vi "CommandDynamixelPositionNoNotifiers.vi"(6 "NotifierReff":T1, 7 "Dynamixel Bounds":T4={"Main Dynamixel Set Data"={"Lower Winch Bound (deg)"=0.0, "Upper Winch Bound (deg)"=800.0}, "Rudder Dynamixel Set Data"={"Lower Winch Bound (deg)"=0.0, "Upper Winch Bound (deg)"=30.0}, "Jib Dynamixel Set Data"={"Lower Winch Bound (deg)"=0.0, "Upper Winch Bound (deg)"=800.0}}, 8 "error in":errorcluster, 9 "FPGA VI Reference In":refnum<k20>, 10 "Dynamixel Cycles":T3, 11 "VISA resource name":refnum<visa-resource-name>) -> (0 "Error out":errorcluster, 2 "Commanded rudder value":T2 min=-0.95 max=0.95 scale=1.0..-1.0, 3 "Debug sail value":dbl, 5 "VISA resource name OUT":refnum<visa-resource-name>)   [LabVIEW 2013]
doc: "First thing to know is that there is a boolean detection switch in this VI that you can switch between RC testing and code control.\n\nWhen RC testing, this VI checks the FPGA for RC data, bounds it so that the data is from 0-1 in steps of 0.05, converts that 0-1 value (or -1 to 1 for the rudder) into Dynamixel degrees (1200 dynamixel counts per 360 degrees) and then writes that position to the Dynamixel. This is highly dependent on the motor bounds which are passed in from above, because a sail value of 1 means different things when the motor bounds are different.\n\nCode control takes the notifier with sail/rudder positions and commands those positions.\n\nEric Schneider, October 2014"
uses:
  Data/TypeDefs/MotorSetup.ctl
  Data/TypeDefs/DynamixelSetupInfo.ctl
  Data/TypeDefs/DynamixelCycleTracker.ctl
  Data/TypeDefs/Rudder Set Suggestions.ctl
  Data/TypeDefs/Notifiers.ctl
  Data/TypeDefs/UTM Location.ctl
  Data/TypeDefs/Sail Set Suggestions.ctl
  Data/TypeDefs/OverrideInformation.ctl
  Data/TypeDefs/OverrideMode.ctl
  Data/TypeDefs/AirmarStatus.ctl
  Data/TypeDefs/HardwareOnline.ctl
  Data/TypeDefs/RC Input Values.ctl
  Classes/Waypoint/Waypoint.lvclass
panel:
  out "Use RC Control?":bool
  out "Rudder written value":dbl
  out "Main written value":dbl
  out "Jib written value":dbl
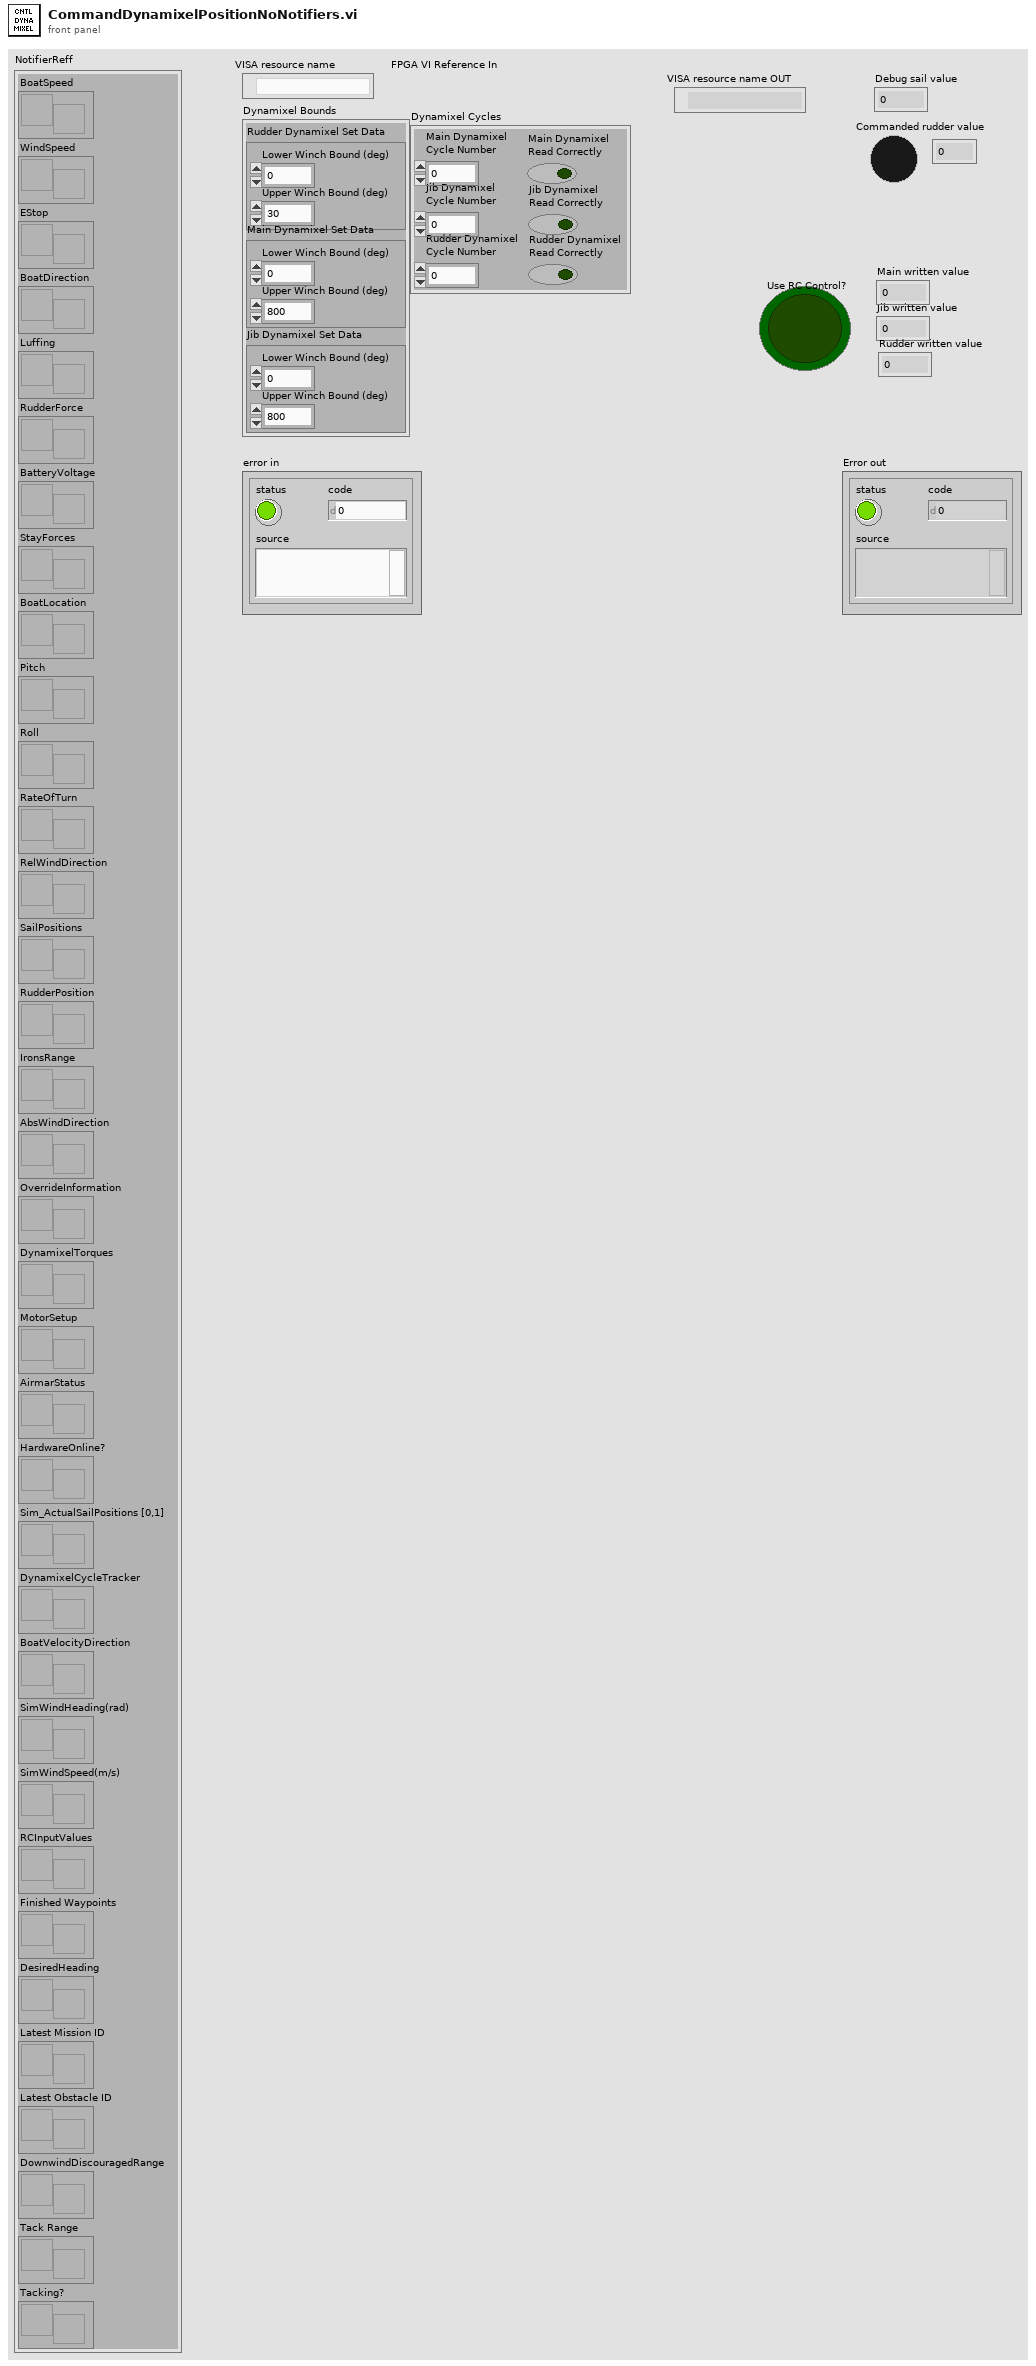
[diagram p1: front panel]
types:
  T1 = typedef "Notifiers.ctl" = cluster{"BoatSpeed":refnum<notifier>, "WindSpeed":refnum<notifier>, "EStop":refnum<notifier>, "BoatDirection":refnum<notifier>, "Luffing":refnum<notifier>, "RudderForce":refnum<notifier>, "BatteryVoltage":refnum<notifier>, "StayForces":refnum<notifier>, "BoatLocation":refnum<notifier>, "Pitch":refnum<notifier>, "Roll":refnum<notifier>, "RateOfTurn":refnum<notifier>, "RelWindDirection":refnum<notifier>, "SailPositions":refnum<notifier>, "RudderPosition":refnum<notifier>, "IronsRange":refnum<notifier>, "AbsWindDirection":refnum<notifier>, "OverrideInformation":refnum<notifier>, "DynamixelTorques":refnum<notifier>, "MotorSetup":refnum<notifier>, "AirmarStatus":refnum<notifier>, "HardwareOnline?":refnum<notifier>, "Sim_ActualSailPositions [0,1]":refnum<notifier>, "DynamixelCycleTracker":refnum<notifier>, "BoatVelocityDirection":refnum<notifier>, "SimWindHeading(rad)":refnum<notifier>, "SimWindSpeed(m/s)":refnum<notifier>, "RCInputValues":refnum<notifier>, "Finished Waypoints":refnum<notifier>, "DesiredHeading":refnum<notifier>, "Latest Mission ID":refnum<notifier>, "Latest Obstacle ID":refnum<notifier>, "DownwindDiscouragedRange":refnum<notifier>, "Tack Range":refnum<notifier>, "Tacking?":refnum<notifier>}
  T2 = typedef "Rudder Set Suggestions.ctl" = dbl
  T3 = typedef "DynamixelCycleTracker.ctl" = cluster{"Main Dynamixel\nCycle Number":i32, "Jib Dynamixel\nCycle Number":i32, "Rudder Dynamixel\nCycle Number":i32, "Main Dynamixel\nRead Correctly":bool, "Jib Dynamixel\nRead Correctly":bool, "Rudder Dynamixel\nRead Correctly":bool}
  T4 = typedef "MotorSetup.ctl" = cluster{"Main Dynamixel Set Data":T5, "Rudder Dynamixel Set Data":T5, "Jib Dynamixel Set Data":T5}
  T5 = typedef "DynamixelSetupInfo.ctl" = cluster{"Lower Winch Bound (deg)":dbl, "Upper Winch Bound (deg)":dbl}
  T6 = typedef "Sail Set Suggestions.ctl" = cluster{"MainSailSuggestion":dbl, "JibSailSuggestion":dbl}
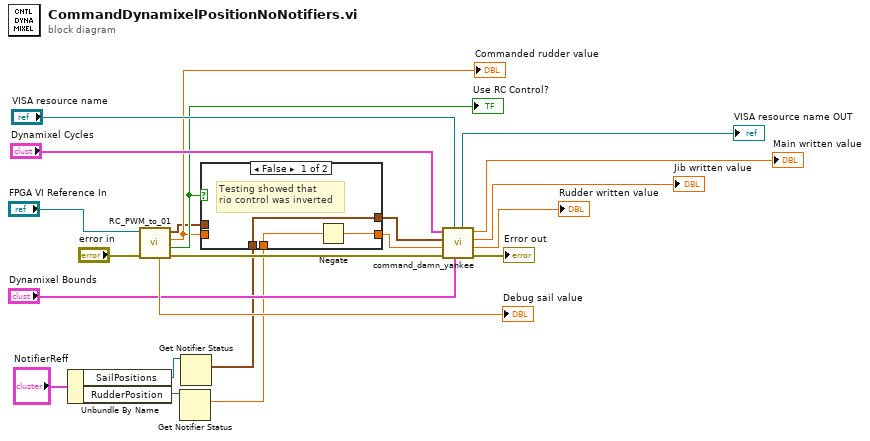
[diagram p0: block diagram]
diagram:
  n1 = Unbundle By Name("NotifierReff") -> ("SailPositions"=w3:refnum<notifier>, "RudderPosition"=w4:refnum<notifier>)
  n2 = call "RC_PWM_to_01.vi"("error in (no error)"="error in", "Refnum in"="FPGA VI Reference In") -> ("error out"=w20:errorcluster, "Use RC Control?"=w10:bool, "Rudder Control Output"=w9:dbl, "Hand Sail Control"=w8:T6, "Sail Debug Output"=→"Debug sail value":dbl)  [unwired: 5 in]
  "Commanded rudder value" <- w9
  "Use RC Control?" <- w10
  n3 = Get Notifier Status(notifier=w4) -> (current notification=w1:T2)  [unwired: 1 in, 4 out]
  n4 = Get Notifier Status(notifier=w3) -> (current notification=w2:T6)  [unwired: 1 in, 4 out]
  n5 = case shown="False" w10 {
    tunnel: w9 -> [_ w27]
    tunnel: w8 -> [_ w26]
    tunnel: [w23 w27] -> w7
    tunnel: [w25 w26] -> w6
    tunnel: w2 -> [w25 _]
    tunnel: w1 -> [w24 _]
    frame False {
      # "Testing showed that\nrio control was inverted"
      n6 = Negate(x=w24) -> (-x=w23:T2)
    }
    frame True {
    }
  }
  n7 = call "command_damn_yankee.vi"("Dynamixel Bounds"="Dynamixel Bounds", "VISA Refnum in"="VISA resource name", "error in (no error)"=w20, "Rudder Control"=w7, "Sail Control"=w6, "Dynamixel Cycles"="Dynamixel Cycles") -> ("error out"=→"Error out":errorcluster, "Rudder written value"=→"Rudder written value":dbl, "Jib written value"=→"Jib written value":dbl, "Main written value"=→"Main written value":dbl, "VISA Refnum out"=→"VISA resource name OUT":refnum<visa-resource-name>)  [unwired: 1 in]
